vi "Read position mMc Edited.vi"(1 "Port":T1={"P type"=0, "reference"="", " Terminator "="\r\n", "Timeout"=300} {"Timeout" step=10; "P type" items=["none", "RS-232C"]}, 3 "error in (no error)":errorcluster, 5 "Controller #":string) -> (6 "Cnt pos":dbl, 7 "Enc pos":dbl, 9 "error out":errorcluster)   [LabVIEW 2021]
panel:
  # "Read position"
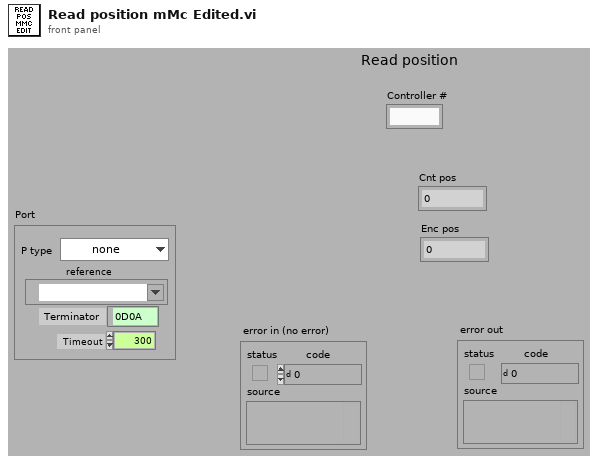
[diagram p1: front panel]
types:
  T1 = cluster{"P type":u16, "reference":refnum<visa-resource-name>, " Terminator ":string, "Timeout":i32}
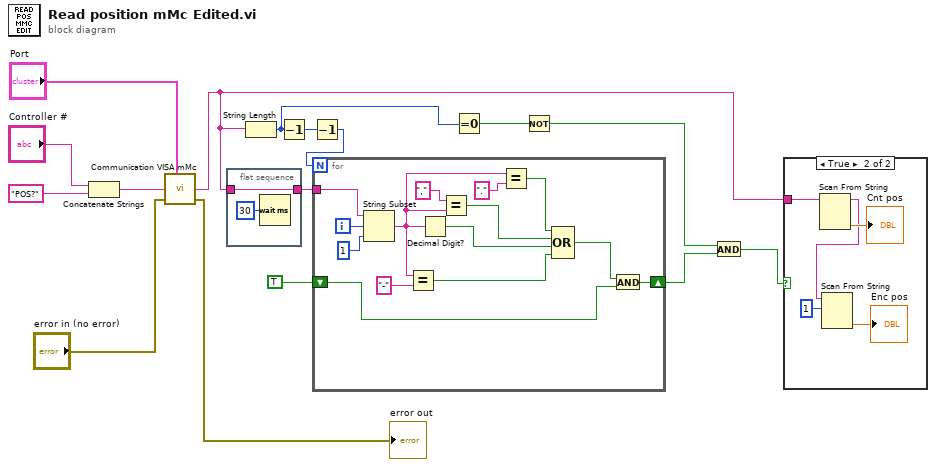
[diagram p0: block diagram]
diagram:
  n1 = Concatenate Strings("Controller #", "POS?") -> (w13:string)
  n2 = call "Communication VISA mMc.vi"("Port"="Port", "Command"=w13, "error in (no error)"="error in (no error)") -> ("Return"=w1:string, "error out"=→"error out":errorcluster)  [unwired: 3 in, 2 out]
  n3 = flat-sequence {
    tunnel: w1 -> [w18]
    tunnel: [w18] -> w2
    frame #0 {
      n4 = Wait (ms)(milliseconds to wait=u32 30) -> ()  [unwired: 1 out]
    }
  }
  n5 = String Length(string=w1) -> (length=w7:i32)
  n6 = Decrement(x=w7) -> (x-1=w8:i32)
  n7 = Decrement(x=w8) -> (x-1=w9:i32)
  n8 = for {
    N: w9 -> [_]
    tunnel: w2 -> [w31]
    shift-right: [w28] -> w5
    shift-left: TRUE -> [w25]
    i -> [w29]
    n9 = String Subset(string=w31, offset (0)=w29, length (rest)=1 ("length (rest)")) -> (substring=w20:string)
    n10 = Equal?(x=w20, y="-") -> (x = y?=w19:bool)
    n11 = Decimal Digit?(1:w20) -> (0:w21:bool)
    n12 = Equal?(x=",", y=w20) -> (x = y?=w22:bool)
    n13 = Equal?(x=w20, y=".") -> (x = y?=w23:bool)
    n14 = Compound Arithmetic op=OR(w23, w22, w21, w19) -> (w24:bool)
    n15 = And(x=w24, y=w25) -> (x .and. y?=w28:bool)
  }
  n16 = Equal To 0?(x=w7) -> (x = 0?=w4:bool)
  n17 = Not(x=w4) -> (.not. x?=w3:bool)
  n18 = And(x=w3, y=w5) -> (x .and. y?=w6:bool)
  n19 = case shown="True" w6 {
    tunnel: w1 -> [_ w36]
    frame False {
    }
    frame True {
      n20 = Scan From String(input string=w36) -> (remaining string=w35:string, output 1=→"Cnt pos":dbl)  [unwired: 4 in, 2 out]
      n21 = Scan From String(input string=w35, initial scan location=u32 1) -> (output 1=→"Enc pos":dbl)  [unwired: 3 in, 3 out]
    }
  }
